vi "Ultrasonic Test.vi"() -> ()   [LabVIEW 2014]
panel:
  out "Distance":dbl
  in  "stop":bool
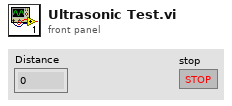
[diagram p1: front panel]
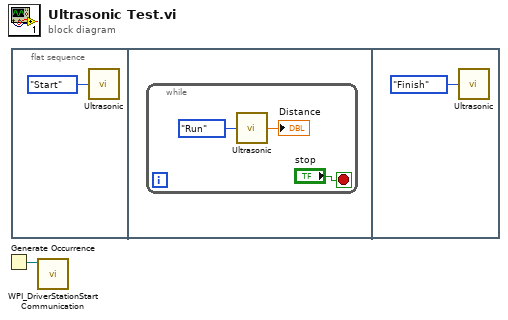
[diagram p0: block diagram]
diagram:
  n1 = Generate Occurrence() -> (w1:refnum<k4>)
  n2 = flat-sequence {
    frame #0 {
      n3 = call "Ultrasonic.vi"("State"=enum8{"Start", "Run", "Finish"}."Start" ("Mode")) -> ()  [unwired: 1 out]
    }
    frame #1 {
      n4 = while {
        stop <- "stop" stop-if-true
        n5 = call "Ultrasonic.vi"("State"=enum8{"Start", "Run", "Finish"}."Run" ("Mode")) -> ("Distance"=→"Distance":dbl)
      }
    }
    frame #2 {
      n6 = call "Ultrasonic.vi"("State"=enum8{"Start", "Run", "Finish"}."Finish" ("Mode")) -> ()  [unwired: 1 out]
    }
  }
  n7 = call <vilib>:"WPI_DriverStationStart Communication.vi"("occurrence"=w1) -> ()  [unwired: 11 in]
